vi "Configure SerDes Script.vi"(7 "verbose? (T)":bool=TRUE, 8 "error in":errorcluster, 9 "scripts":path[](array[path]), 10 "bus instance names":string[](array[string]), 11 "FPGA Ref In":refnum<k20>) -> (0 "error out":errorcluster, 2 "outputs":string[](array[string]), 3 "FPGA Ref Out":refnum<k20>)   [LabVIEW 2025, in "I2C Bus Monitor.lvclass"]
uses:
  I2C Bus Monitor.lvclass
  <instrlib>/FlexRIO/API/Host/v1/NI FlexRIO API v1.lvlib
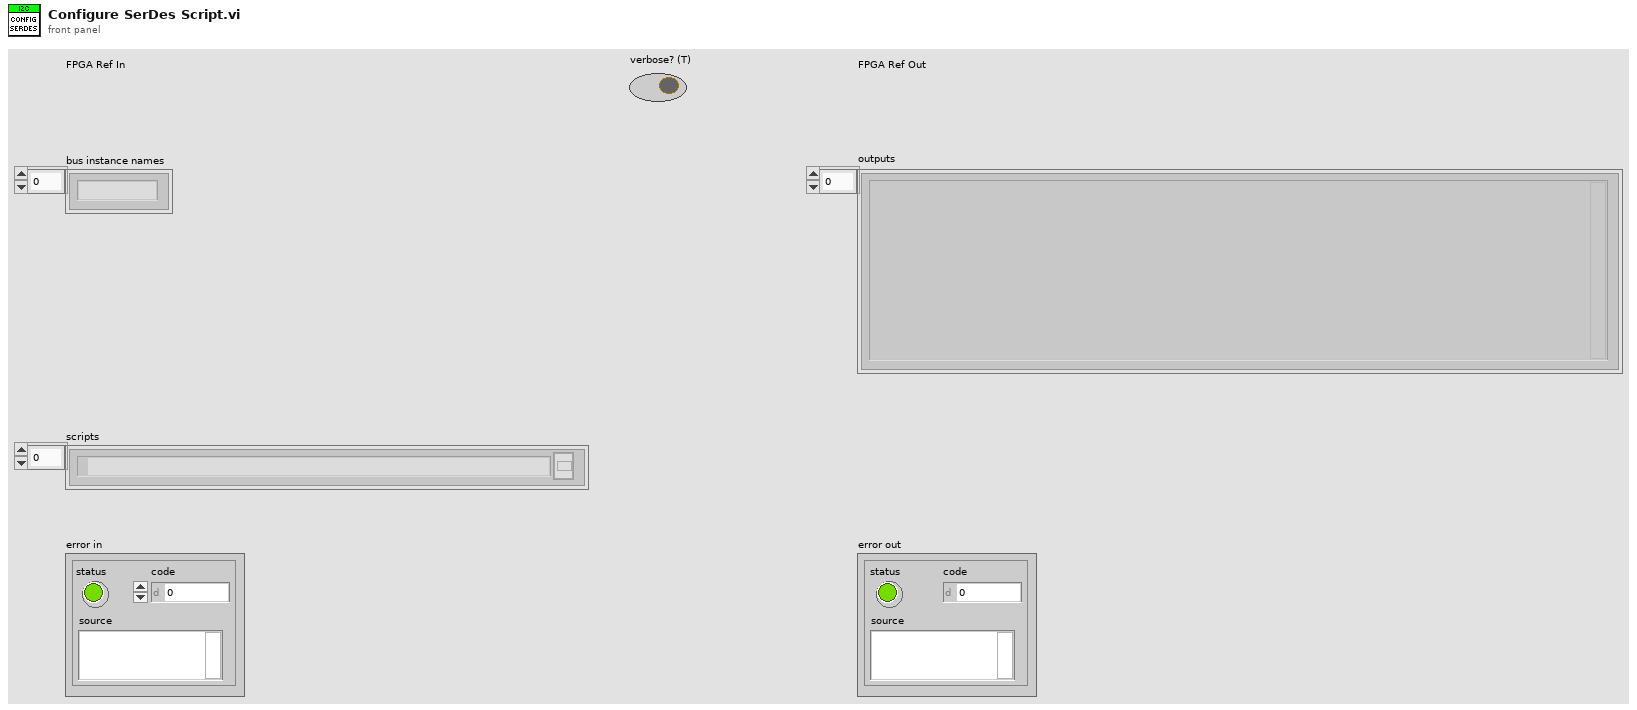
[diagram p1: front panel]
types:
  T1 = enum16{"open", "replace", "create", "open or create", "replace or create", "replace or create with confirmation"}
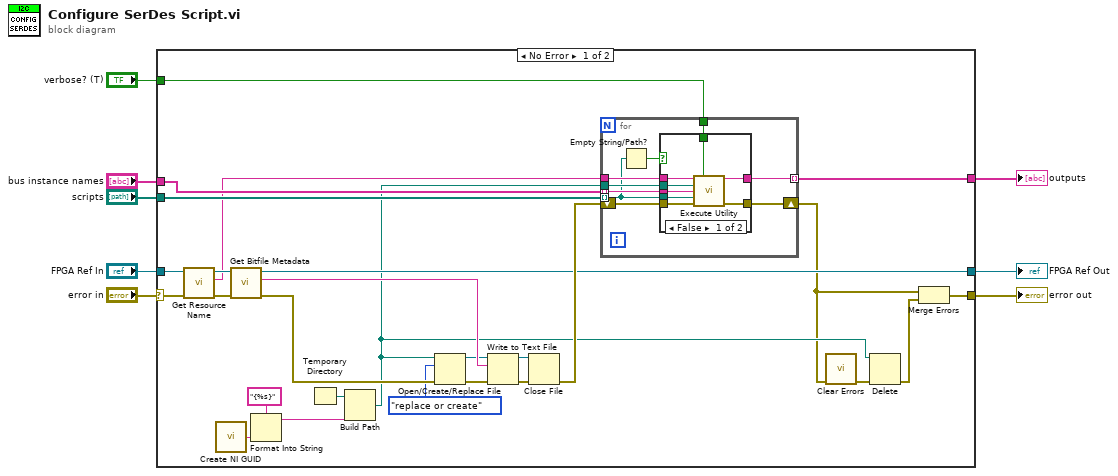
[diagram p0: block diagram]
diagram:
  n1 = case shown="No Error" "error in" {
    selector: "error in" -> [w23 w55]
    tunnel: "bus instance names" -> [w28 _]
    tunnel: "scripts" -> [w27 _]
    tunnel: "FPGA Ref In" -> [w25 w54]
    tunnel: "verbose? (T)" -> [w21 _]
    tunnel: [w20 _] -> w3
    tunnel: [w19 w54] -> w2
    tunnel: [w12 w55] -> w1
    frame No Error {
      n2 = call "Get Resource Name.vi"("error in"=w23, "FPGA Ref In"=w25) -> ("error out"=w24:errorcluster, "resource name"=w18:string, "FPGA Ref Out"=w22:refnum<k20>)  [unwired: 6 in, 1 out]
      n3 = call <vilib>:"Create NI GUID.vi"() -> ("NI GUID"=w10:string)
      n4 = call <instrlib>:"Get Bitfile Metadata.vi"("error in"=w24, "fpga interface in"=w22) -> ("error out"=w35:errorcluster, "metadata"=w34:string, "fpga interface out"=w19:refnum<k20>)  [unwired: 7 in]
      n5 = Format Into String(format string="{%s}" ("name or relative path"), w10) -> (resulting string=w9:string)  [unwired: 2 in, 1 out]
      n6 = Temporary Directory() -> (w17:path)
      n7 = Build Path(base path=w17, name or relative path=w9) -> (appended path=w16:path)
      n8 = Open/Create/Replace File(file path (use dialog)=w16, error in=w35, operation (0:open)=T1."replace or create") -> (refnum out=w32:refnum<file>, error out=w33:errorcluster)  [unwired: 3 in, 1 out]
      n9 = Write to Text File(file (use dialog)=w32, text=w34, error in=w33) -> (refnum out=w30:refnum<file>, error out=w31:errorcluster)  [unwired: 1 in, 1 out]
      n10 = Close File(refnum=w30, error in=w31) -> (error out=w26:errorcluster)  [unwired: 1 out]
      n11 = for {
        tunnel: w28 -> [w44] mode=indexing
        tunnel: w27 -> [w36] mode=indexing
        tunnel: w21 -> [w42]
        tunnel: [w41] -> w20 mode=indexing
        tunnel: w18 -> [w40]
        tunnel: w16 -> [w39]
        shift-right: [w38] -> w14
        shift-left: w26 -> [w43]
        n12 = Empty String/Path?(string/path=w36) -> (empty?=w37:bool)
        n13 = case shown="False" w37 {
          tunnel: w44 -> [w52 _]
          tunnel: w36 -> [w51 _]
          tunnel: w43 -> [w50 w53]
          tunnel: w42 -> [w49 _]
          tunnel: [w48 _] -> w41
          tunnel: w40 -> [w47 _]
          tunnel: w39 -> [w46 _]
          tunnel: [w45 w53] -> w38
          frame False {
            n14 = call "Execute Utility.vi"("resource"=w47, "verbose?"=w49, "bitfile"=w46, "serdes"=w52, "script"=w51, "error in"=w50) -> ("standard output"=w48:string, "error out"=w45:errorcluster)  [unwired: 6 in, 2 out]
          }
          frame True {
          }
        }
      }
      n15 = call <vilib>:"Clear Errors.vi"("error in (no error)"=w14) -> ("error out"=w15:errorcluster)  [unwired: 5 in, 1 out]
      n16 = Delete(path (use dialog)=w16, error in=w15) -> (error out=w13:errorcluster)  [unwired: 3 in, 2 out]
      n17 = Merge Errors(w14, w13) -> (w12:errorcluster)
    }
    frame Error {
    }
  }
  "FPGA Ref Out" <- w2
  "error out" <- w1
  "outputs" <- w3
